vi "voltage without drive coil times.vi"(8 "error in (no error)":errorcluster, 11 "display queues":T2) -> (0 "error out":errorcluster, 2 "not currently in coil veto":bool, 3 "voltage_no_coil":T1[](array[typedef]))   [LabVIEW 2017]
uses:
  typedefs/queue cluster.ctl
  typedefs/reading1.ctl
  typedefs/reading3.ctl
panel:
  out "votl time in min":dbl
  out "volt time in max":dbl
  out "coil min":dbl
  out "coil max":dbl
  out "min value":dbl
  out "max value":dbl
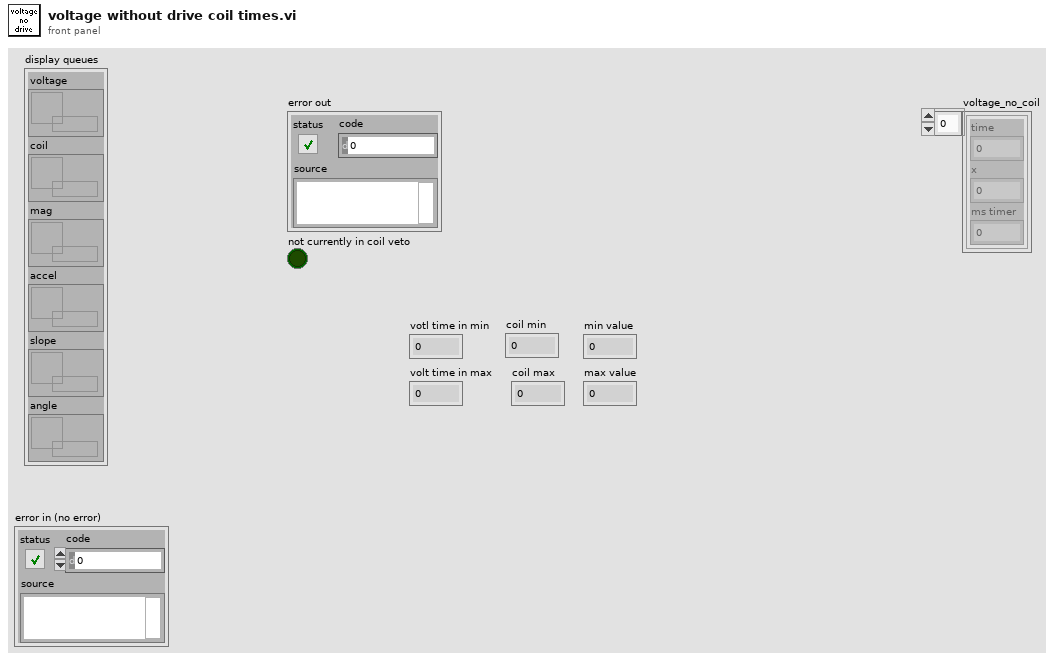
[diagram p1: front panel]
types:
  T1 = typedef "reading1.ctl" = cluster{"time":dbl, "x":dbl, "ms timer":u32}
  T2 = typedef "queue cluster.ctl" = cluster{"voltage":refnum<queue>, "coil":refnum<queue>, "mag":refnum<queue>, "accel":refnum<queue>, "slope":refnum<queue>, "angle":refnum<queue>}
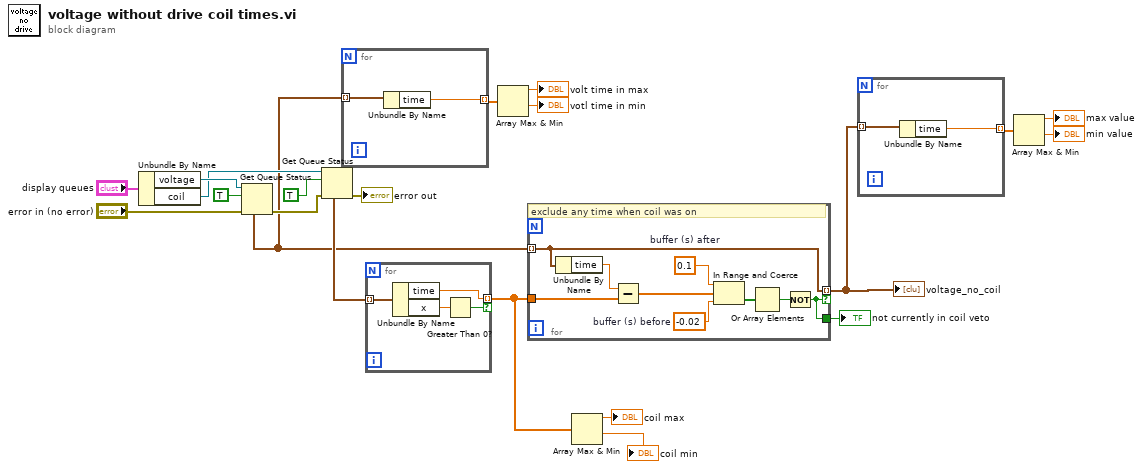
[diagram p0: block diagram]
diagram:
  n1 = Unbundle By Name("display queues") -> ("voltage"=w21:refnum<queue>, "coil"=w18:refnum<queue>)
  n2 = Get Queue Status(queue=w21, return elements? (F)=TRUE, error in (no error)="error in (no error)") -> (error out=w17:errorcluster, elements=w1:T1[])  [unwired: 6 out]
  n3 = Get Queue Status(queue=w18, return elements? (F)=TRUE, error in (no error)=w17) -> (error out=→"error out":errorcluster, elements=w15:T1[])  [unwired: 6 out]
  n4 = for {
    tunnel: w1 -> [w23] mode=indexing
    tunnel: [w22] -> w4 mode=indexing
    n5 = Unbundle By Name(w23) -> ("time"=w22:dbl)
  }
  n6 = for {
    tunnel: w15 -> [w26] mode=indexing
    tunnel: [w24] -> w7 mode=indexing if=w25
    n7 = Unbundle By Name(w26) -> ("time"=w24:dbl, "x"=w27:dbl)
    n8 = Greater Than 0?(x=w27) -> (x > 0?=w25:bool)
  }
  n9 = Array Max & Min(array=w4) -> (max value=→"volt time in max":dbl, min value=→"votl time in min":dbl)  [unwired: 2 out]
  n10 = for {
    tunnel: w1 -> [w36] mode=indexing
    tunnel: [w36] -> w11 mode=indexing if=w28
    tunnel: w7 -> [w34]
    tunnel: [w28] -> w12
    w31 = -0.02  # buffer (s) before
    w32 = 0.1  # buffer (s) after
    # "exclude any time when coil was on"
    n11 = Unbundle By Name(w36) -> ("time"=w35:dbl)
    n12 = Subtract(x=w35, y=w34) -> (x-y=w33:dbl[])
    n13 = In Range and Coerce(upper limit=w32, x=w33, lower limit=w31) -> (In Range?=w30:bool[])  [unwired: 1 out]
    n14 = Or Array Elements(Boolean array=w30) -> (logical OR=w29:bool)
    n15 = Not(x=w29) -> (.not. x?=w28:bool)
  }
  "voltage_no_coil" <- w11
  "not currently in coil veto" <- w12
  n16 = Array Max & Min(array=w7) -> (max value=→"coil max":dbl, min value=→"coil min":dbl)  [unwired: 2 out]
  n17 = for {
    tunnel: w11 -> [w38] mode=indexing
    tunnel: [w37] -> w10 mode=indexing
    n18 = Unbundle By Name(w38) -> ("time"=w37:dbl)
  }
  n19 = Array Max & Min(array=w10) -> (max value=→"max value":dbl, min value=→"min value":dbl)  [unwired: 2 out]
